vi "getPressure.vi"(6 "Channel":i32, 8 "error in (no error)":errorcluster, 11 "Instrument.Cryostat in":refnum<class "Instrument.Cryostat.lvclass">) -> (0 "error out":errorcluster, 1 "Status":string, 2 "Pressure (mbar)":dbl, 3 "Instrument.Cryostat out":refnum<class "Instrument.Cryostat.lvclass">)   [LabVIEW 2019, in "Instrument.Cryostat.lvclass"]
uses:
  Instrument.Cryostat.lvclass
  C:/Users/patrick/Documents/GitHub/Instrument-Framework/lvsrc/Instrument/Instrument.lvclass
  Typedefs/getPressure--cluster.ctl
  Typedefs/Cryostat.commands--enum.ctl
  21f7b314-a6ba-4151-b6ad-b7a5cd4b84b8.vi
  21f7b314-a6ba-4151-b6ad-b7a5cd4b84b8.vi/51f0ecac-9e3e-49b6-8cc9-4ab80f94526b.vi
  21f7b314-a6ba-4151-b6ad-b7a5cd4b84b8.vi/51f0ecac-9e3e-49b6-8cc9-4ab80f94526b.vi/a449e028-28cc-408a-9ee1-380c6c6e30ee.vi
  21f7b314-a6ba-4151-b6ad-b7a5cd4b84b8.vi/51f0ecac-9e3e-49b6-8cc9-4ab80f94526b.vi/98e218ba-e1b6-4119-b8c4-b6fedf715667.vi
  Instrument/Protected/Validate API method.vi
  Instrument/Private/Get RC Connection Status.vi
  Instrument/API/Send and Receive.vi
  <vilib>/Utility/Data Type/Get Type Information.vi
  <vilib>/JDP Science/JSONtext/JSON text to Variant.vi
  <vilib>/JDP Science/JSONtext/LVClass Serializer/JSONtext LVClass Serializer.lvclass
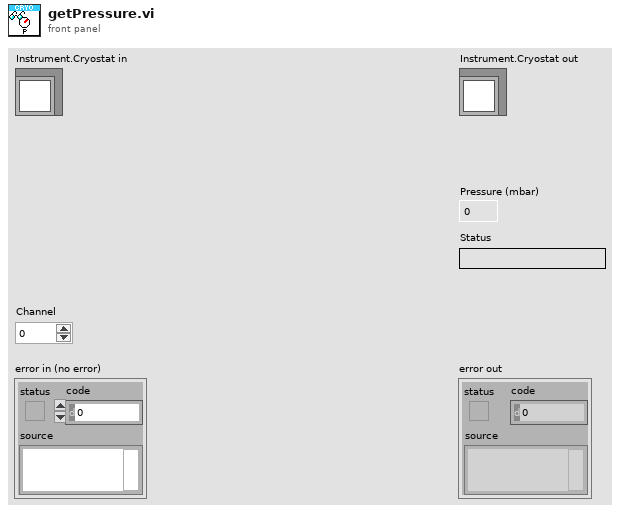
[diagram p1: front panel]
types:
  T1 = typedef "Instrument.Cryostat.lvclass/Cryostat.commands--enum.ctl" = enum16{"getLN2Level", "getLHeLevel", "getMagnet", "getMagnetVector", "setMagnet", "setMagnetVector", "getAngle", "setAngle", "getTemperature", "setTemperature", "getHeater", "setHeater", "getChamber", "setChamber", "getPressure"}
  T2 = typedef "Instrument.Cryostat.lvclass/getPressure--cluster.ctl" = cluster{"pressure":dbl, "status":string}
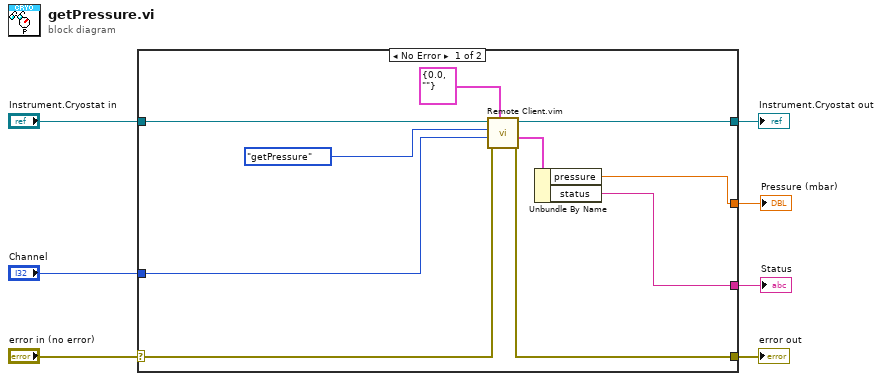
[diagram p0: block diagram]
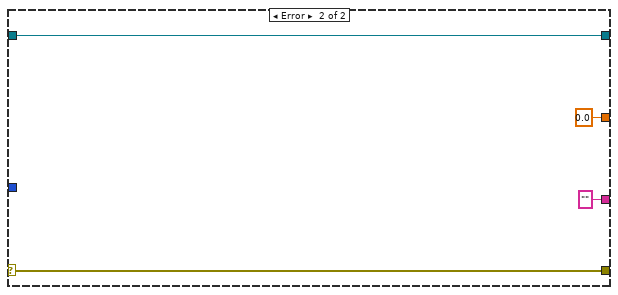
[diagram p2: hidden frame]
diagram:
  n1 = case shown="No Error" "error in (no error)" {
    selector: "error in (no error)" -> [w8 w21]
    tunnel: [w15 w21] -> w6
    tunnel: [w17 w20] -> w4
    tunnel: "Instrument.Cryostat in" -> [w9 w20]
    tunnel: "Channel" -> [w16 _]
    tunnel: [w13 0.0 ("Pressure")] -> w2
    tunnel: [w12 "" ("Status")] -> w1
    frame No Error {
      n2 = call "Remote Client.vim"("Data Out type"=T2 {"pressure"=0.0, "status"=""} ("getPressure"), "error in (no error)"=w8, "Data in"=w16, "Command in"=Cryostat.commands--enum."getPressure" ("commands"), "Instrument in"=w9) -> ("error out"=w15:errorcluster, "Data out"=w14:T2, "Instrument out"=w17:refnum<class "Instrument.Cryostat.lvclass">)  [unwired: 3 in, 1 out]
      n3 = Unbundle By Name(w14) -> ("pressure"=w13:dbl, "status"=w12:string)
    }
    frame Error {
    }
  }
  "error out" <- w6
  "Instrument.Cryostat out" <- w4
  "Pressure (mbar)" <- w2
  "Status" <- w1
